vi "CMDSendToQueue.vi"(9 "arg2":u16, 10 "arg1":u16, 11 "CMD":i8) -> ()   [LabVIEW 2017]
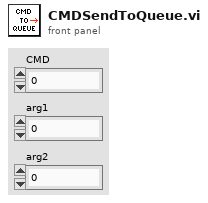
[diagram p1: front panel]
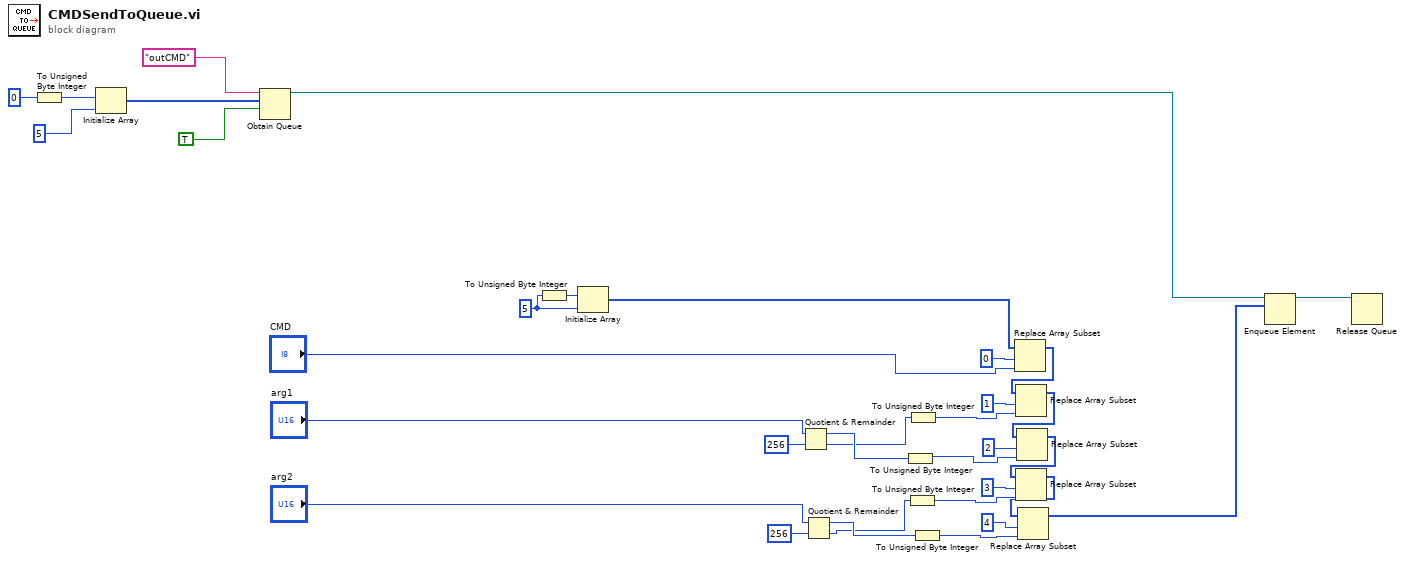
[diagram p0: block diagram]
diagram:
  w11 = 5 ("dimension size")
  n1 = To Unsigned Byte Integer(number=u8 0) -> (unsigned 8bit integer=w8:u8)
  n2 = Initialize Array(w8, 5 ("dimension size")) -> (w5:u8[])
  n3 = Obtain Queue(name (unnamed)="outCMD", element data type=w5, create if not found? (T)=TRUE) -> (queue out=w3:refnum<queue>)  [unwired: 2 in, 2 out]
  n4 = To Unsigned Byte Integer(number=w11) -> (unsigned 8bit integer=w12:u8)
  n5 = Initialize Array(w12, w11) -> (w10:u8[])
  n6 = Quotient & Remainder(x="arg1", y=i16 256) -> (x-y*floor(x/y)=w20:u16, floor(x/y)=w19:u16)
  n7 = Quotient & Remainder(x="arg2", y=i16 256) -> (x-y*floor(x/y)=w18:u16, floor(x/y)=w17:u16)
  n8 = To Unsigned Byte Integer(number=w20) -> (unsigned 8bit integer=w27:u8)
  n9 = To Unsigned Byte Integer(number=w17) -> (unsigned 8bit integer=w26:u8)
  n10 = To Unsigned Byte Integer(number=w19) -> (unsigned 8bit integer=w28:u8)
  n11 = To Unsigned Byte Integer(number=w18) -> (unsigned 8bit integer=w25:u8)
  n12 = Replace Array Subset(array=w10, new element="CMD", index=0) -> (w16:u8[])
  n13 = Replace Array Subset(array=w16, new element=w28, index=1) -> (w15:u8[])
  n14 = Replace Array Subset(array=w15, new element=w27, index=2) -> (w14:u8[])
  n15 = Replace Array Subset(array=w14, new element=w26, index=3) -> (w13:u8[])
  n16 = Replace Array Subset(array=w13, new element=w25, index=4) -> (w2:u8[])
  n17 = Enqueue Element(queue=w3, element=w2) -> (queue out=w1:refnum<queue>)  [unwired: 2 in, 2 out]
  n18 = Release Queue(queue=w1) -> ()  [unwired: 2 in, 3 out]
